vi "locate enable channel.vi"(8 "error in":errorcluster, 11 "TDMS datalogger editor node in":refnum<class "TDMS datalogger editor node.lvclass">) -> (0 "error out":errorcluster, 1 "channel":refnum<class "TBM channel.lvclass">, 2 "Tag Name":string, 3 "TDMS datalogger editor node out":refnum<class "TDMS datalogger editor node.lvclass">)   [LabVIEW 2013, in "TDMS datalogger editor node.lvclass"]
uses:
  TDMS datalogger editor node.lvclass
  <vilib>/NI/TBM Modules/TDMS Datalogger/module/configuration/TDMS datalogger configuration.lvclass
  <vilib>/NI/Tag Bus Module Framework/channel/TBM channel.lvclass
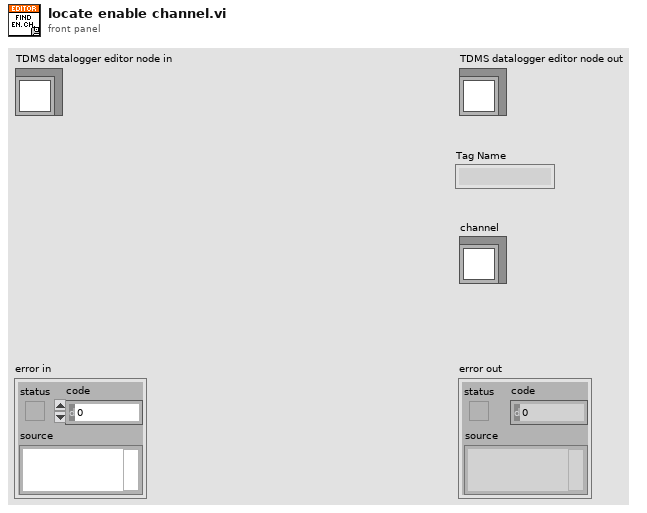
[diagram p1: front panel]
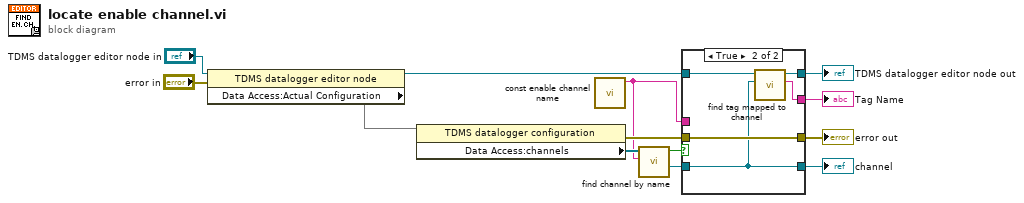
[diagram p0: block diagram]
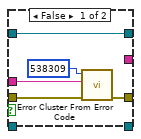
[diagram p2: hidden frame]
diagram:
  n1 = property class="TDMS datalogger editor node"(reference="TDMS datalogger editor node in", error in="error in") -> (reference out=w7:refnum<class "TDMS datalogger editor node.lvclass">, "Data Access:Actual Configuration"=w11)  [unwired: 1 out]
  n2 = property class="TDMS datalogger configuration"(reference=w11) -> (error out=w3:errorcluster, "Data Access:channels"=w10:refnum<class "TBM channel.lvclass">[])  [unwired: 1 in, 1 out]
  n3 = call <vilib>:"const enable channel name.vi"() -> ("enable channel"=w2:string)  [unwired: 11 in]
  n4 = call <vilib>:"find channel by name.vi"("channel name"=w2, "channel list"=w10) -> ("channel duplicate"=w8:refnum<class "TBM channel.lvclass">, "found?"=w9:bool)  [unwired: 7 in, 1 out]
  n5 = case shown="True" w9 {
    tunnel: w8 -> [_ w19]
    tunnel: w7 -> [w18 w23]
    tunnel: [w18 w22] -> w6
    tunnel: [_ w21] -> w5
    tunnel: [_ w19] -> w4
    tunnel: w3 -> [w15 w20]
    tunnel: w2 -> [w17 _]
    tunnel: [w14 w20] -> w1
    frame False {
      n6 = call <vilib>:"Error Cluster From Error Code.vi"("error in (no error)"=w15, "error message (\"\")"=w17, "error code (0)"=538309) -> ("error out"=w14:errorcluster)  [unwired: 6 in]
    }
    frame True {
      n7 = call <vilib>:"find tag mapped to channel.vi"("TBM channel"=w19, "module editor node in"=w23) -> ("Tag Name"=w21:string, "module editor node out"=w22:refnum<class "TDMS datalogger editor node.lvclass">)  [unwired: 8 in]
    }
  }
  "error out" <- w1
  "TDMS datalogger editor node out" <- w6
  "Tag Name" <- w5
  "channel" <- w4
